vi "REV2_Read_Pack.vi"(8 "error in (no error)":errorcluster, 11 "VISA Refnum in":refnum<visa-resource-name>) -> (0 "error out":errorcluster, 2 "output cluster":T1, 3 "VISA Refnum out":refnum<visa-resource-name>)   [LabVIEW 2016, in "REV_2.lvlib"]
uses:
  REV_2.lvlib
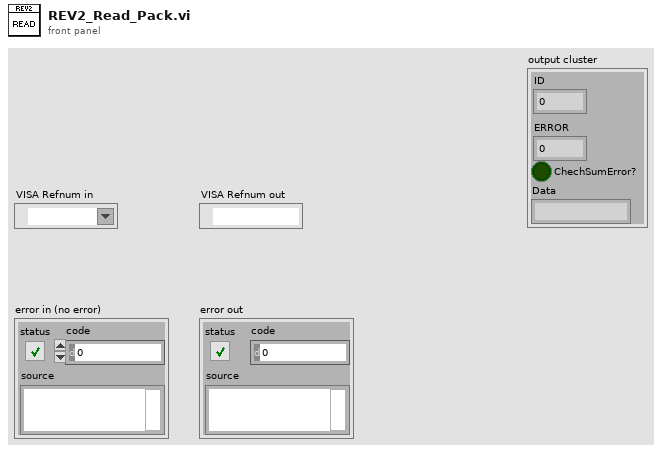
[diagram p1: front panel]
types:
  T1 = cluster{"ID":u8, "ERROR":u8, "ChechSumError?":bool, "Data":string}
  T2 = enum16{"big-endian, network order", "native, host order", "little-endian"}
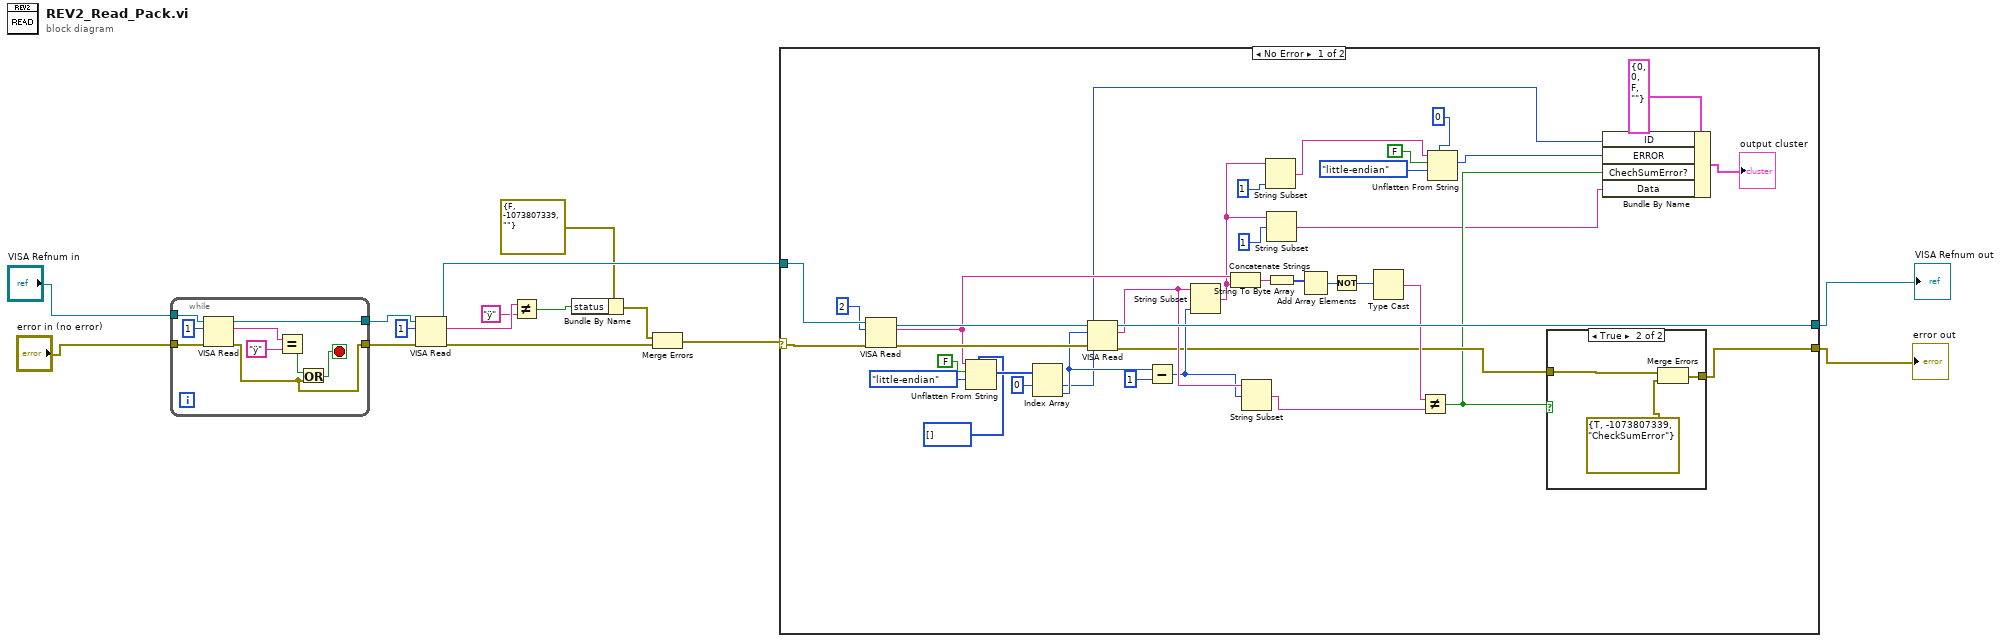
[diagram p0: block diagram]
diagram:
  n1 = while {
    tunnel: [w19] -> w11
    tunnel: "error in (no error)" -> [w18]
    tunnel: "VISA Refnum in" -> [w17]
    tunnel: [w16] -> w10
    stop <- w21 stop-if-true
    n2 = VISA Read(VISA resource name=w17, byte count=u32 1, error in (no error)=w18) -> (VISA resource name out=w16:refnum<visa-resource-name>, read buffer=w23:string, error out=w19:errorcluster)  [unwired: 1 out]
    n3 = Equal?(x=w23, y="ÿ") -> (x = y?=w20:bool)
    n4 = Or(x=w20, y=w19) -> (x .or. y?=w21:bool)
  }
  n5 = VISA Read(VISA resource name=w10, byte count=u32 1, error in (no error)=w11) -> (VISA resource name out=w12:refnum<visa-resource-name>, read buffer=w6:string, error out=w13:errorcluster)  [unwired: 1 out]
  n6 = Not Equal?(x=w6, y="ÿ") -> (x != y?=w3:bool)
  n7 = Bundle By Name(cluster=errorcluster {"status"=FALSE, "code"=-1073807339, "source"=""} ("error constant"), "status"=w3) -> (w2:errorcluster)
  n8 = Merge Errors(w2, w13) -> (w1:errorcluster)
  n9 = case shown="No Error" w1 {
    selector: w1 -> [w51 w66]
    tunnel: [w61 w67] -> w15
    tunnel: [w31 w66] -> w14
    tunnel: w12 -> [w53 w67]
    frame No Error {
      n10 = VISA Read(VISA resource name=w53, byte count=u32 2, error in (no error)=w51) -> (VISA resource name out=w58:refnum<visa-resource-name>, read buffer=w48:string, error out=w57:errorcluster)  [unwired: 1 out]
      n11 = Unflatten From String(type=u8[] [], binary string=w48, data includes array or string size? (T)=FALSE, byte order (0:big-endian, network order)=T2."little-endian") -> (value=w59:u8[])  [unwired: 1 in, 2 out]
      n12 = Index Array(array=w59, index #1=0 ("index")) -> (element #1=w27:u8, element #2=w50:u8)  [unwired: 1 in]
      n13 = VISA Read(VISA resource name=w58, byte count=w50, error in (no error)=w57) -> (VISA resource name out=w61:refnum<visa-resource-name>, read buffer=w43:string, error out=w32:errorcluster)  [unwired: 1 out]
      n14 = Subtract(x=w50, y=u8 1) -> (x-y=w42:u8)
      n15 = String Subset(string=w43, length (rest)=w42) -> (substring=w37:string)  [unwired: 1 in]
      n16 = Concatenate Strings(w48, w37) -> (w45:string)
      n17 = String Subset(string=w43, offset (0)=w42) -> (substring=w41:string)  [unwired: 1 in]
      n18 = String Subset(string=w37, length (rest)=u8 1 ("y")) -> (substring=w34:string)  [unwired: 1 in]
      n19 = String Subset(string=w37, offset (0)=u8 1 ("y")) -> (substring=w25:string)  [unwired: 1 in]
      n20 = String To Byte Array(string=w45) -> (unsigned byte array=w46:u8[])
      n21 = Add Array Elements(numeric array=w46) -> (sum=w47:u8)
      n22 = Not(x=w47) -> (.not. x?=w44:u8)
      n23 = Type Cast(x=w44) -> (*(type *) &x=w40:string)  [unwired: 1 in]
      n24 = Not Equal?(x=w40, y=w41) -> (x != y?=w29:bool)
      n25 = Unflatten From String(type=u8 0 ("y"), binary string=w34, data includes array or string size? (T)=FALSE, byte order (0:big-endian, network order)=T2."little-endian") -> (value=w30:u8)  [unwired: 1 in, 2 out]
      n26 = case shown="True" w29 {
        tunnel: w32 -> [w62 w65]
        tunnel: [w62 w63] -> w31
        frame False {
        }
        frame True {
          n27 = Merge Errors(w65, errorcluster {"status"=TRUE, "code"=-1073807339, "source"="CheckSumError"} ("error constant")) -> (w63:errorcluster)
        }
      }
      n28 = Bundle By Name(cluster=T1 {"ID"=0, "ERROR"=0, "ChechSumError?"=FALSE, "Data"=""} ("output cluster"), "ID"=w27, "ERROR"=w30, "ChechSumError?"=w29, "Data"=w25) -> (→"output cluster":T1)
    }
    frame Error {
    }
  }
  "VISA Refnum out" <- w15
  "error out" <- w14
